vi "FR GUI Measurement setup.vi"(9 "FFmeter settings":T1={"AC Source"={"AC Source type"=enum."Fluke 5XXX calibrator", "VISA"="", "Ref. clock (Hz)"=0.0, "status ref"=refnum}, "TWM pipe"="\\\\.\\pipe\\TWM:server", "Measurement status ref"=refnum, "TWM Status ref"=refnum, "Abort ref"=refnum, "DC meter"={"DC meter type"=enum."H/A/K 3458", "DC meter VISA"="", "NPLC"=10, "status ref"=refnum}, "Measurement properties"={"Measurement frequencies (Hz)"=[1000.0], "Sampling frequency (Hz)"=500000.0, "Signal amplitude (V)"=4.5, "AC-DC settle time (s)"=20.0, "Record length (multiples of period)"=[1000.0, 10000.0, 1000.0], "Measurement template file"=path "", "Row of START keyword"=1, "Row of STOP keyword"=0, "Calculate RMS from samples"=FALSE, "AC-DC warm up time (s)"=300.0, "Measurement template line"=[], "DC meter readings No."=10, "Algorithm"="TWM-WFFT"}, "Skip waiting ref"=refnum, "Octave paths"={"GNU Octave path"=path "C:/Program Files/GNU Octave/Octave-6.2.0/mingw64/bin", "TWM+QWTB path"=path "C:/Users/labina/Desktop/TWM-1.8.7.0-full/octprog", "lvlib path"=path "D:/martin/WAC/WACsw - github/control_software/Filter function meter/external libraries/GOLPI 0.7.3.1 source distribution LV 20.0 32 bit/lv_proc.dll"}, "Template definition"={"Keywords column"=0, "Sig. freq. column"=1, "Rec. len. column"=2, "Meas. points. row min to read"=9, "Meas. points. row max to read"=1509, "Properties column"=4, "Properties row start"=1, "Properties row end"=5, "Keyword START regexp"="", "Keyword STOP regexp"="", "HW data column"=7, "HW data row start"=1, "HW data row end"=3, "TIme and date column start"=3, "Digitizer value column start "=4, "DC mean column start "=6, "DC readings column start"=10}} {"Measurement properties"."Record length (multiples of period)" format="%#_3p"; "Measurement properties"."Sampling frequency (Hz)" format="%#_3p"; "Measurement properties"."Measurement frequencies (Hz)" format="%#_3p"}) -> (3 "FFmeter settings out":T1={"AC Source"={"AC Source type"=enum."Fluke 5XXX calibrator", "VISA"="", "Ref. clock (Hz)"=0.0, "status ref"=refnum}, "TWM pipe"="\\\\.\\pipe\\TWM:server", "Measurement status ref"=refnum, "TWM Status ref"=refnum, "Abort ref"=refnum, "DC meter"={"DC meter type"=enum."H/A/K 3458", "DC meter VISA"="", "NPLC"=10, "status ref"=refnum}, "Measurement properties"={"Measurement frequencies (Hz)"=[1000.0], "Sampling frequency (Hz)"=500000.0, "Signal amplitude (V)"=4.5, "AC-DC settle time (s)"=20.0, "Record length (multiples of period)"=[1000.0, 10000.0, 1000.0], "Measurement template file"=path "", "Row of START keyword"=1, "Row of STOP keyword"=0, "Calculate RMS from samples"=FALSE, "AC-DC warm up time (s)"=300.0, "Measurement template line"=[], "DC meter readings No."=10, "Algorithm"="TWM-WFFT"}, "Skip waiting ref"=refnum, "Octave paths"={"GNU Octave path"=path "C:/Program Files/GNU Octave/Octave-6.2.0/mingw64/bin", "TWM+QWTB path"=path "C:/Users/labina/Desktop/TWM-1.8.7.0-full/octprog", "lvlib path"=path "D:/martin/WAC/WACsw - github/control_software/Filter function meter/external libraries/GOLPI 0.7.3.1 source distribution LV 20.0 32 bit/lv_proc.dll"}, "Template definition"={"Keywords column"=0, "Sig. freq. column"=1, "Rec. len. column"=2, "Meas. points. row min to read"=9, "Meas. points. row max to read"=1509, "Properties column"=4, "Properties row start"=1, "Properties row end"=5, "Keyword START regexp"="", "Keyword STOP regexp"="", "HW data column"=7, "HW data row start"=1, "HW data row end"=3, "TIme and date column start"=3, "Digitizer value column start "=4, "DC mean column start "=6, "DC readings column start"=10}} {"Measurement properties"."Record length (multiples of period)" format="%#_3p"; "Measurement properties"."Sampling frequency (Hz)" format="%#_3p"; "Measurement properties"."Measurement frequencies (Hz)" format="%#_3p"})   [LabVIEW 2020]
uses:
  Type definitions/FFmeter settings.ctl
  General AC source/Type definitions/AC Source.ctl
  General AC source/Type definitions/AC Source type.ctl
  General DC meter/Type definitions/DC meter.ctl
  General DC meter/Type definitions/DC meter type.ctl
  FR Measurement/Type definitions/FR Measuement properties.ctl
  FR Utilities/Type definitions/FR Template definition.ctl
  <vilib>/Utility/error.llb/Error Cluster From Error Code.vi
  <vilib>/ErrorRing/Error Ring.xnode
  external libraries/varilib/varilib.lvlib
panel:
  out "Algorithm":string
  out "dc meter readings":i32=50000 caption="DC meter readings"
  in  "recalculate template":bool
  out "ac-dc warmup time":dbl=50000.0 caption="AC-DC warm-up time" format="%#_6p"
  out "Estimate as formatted text":string
  out "Meas points":i32=1 caption="Measurement points"
  in  "Calculate RMS\nfrom samples":bool
  out "ac-dc settle time":dbl=50000.0 caption="AC-DC settle time" format="%#_6p"
  out "Measurement freq. (Hz) | Record length (periods)":dbl[][](array[numeric])=[[1000.0]] format="%#_3p"
  in  "load template":bool
  in  "Measurement template file":path
  in  "show connections":bool
  out "Signal amplitude (V)":dbl=1.0 caption="AC voltage amplitude"
  out "Sampling frequency (Hz)":dbl=50000.0 caption="Sampling frequency" format="%#_6p"
  out "gui_elements":refnum<vi>[](array[refnum])
  in  "save_and_quit":bool
  in  "cancel":bool
  # "Load the template and check loaded values here:"
  # "s"
  # "V"
  # "Who will make\nnice pictures?\n\nconnection setup here"
  # "Hz"
  # "s"
  # "Who will make\nnice pictures?\n\nwaveforms here"
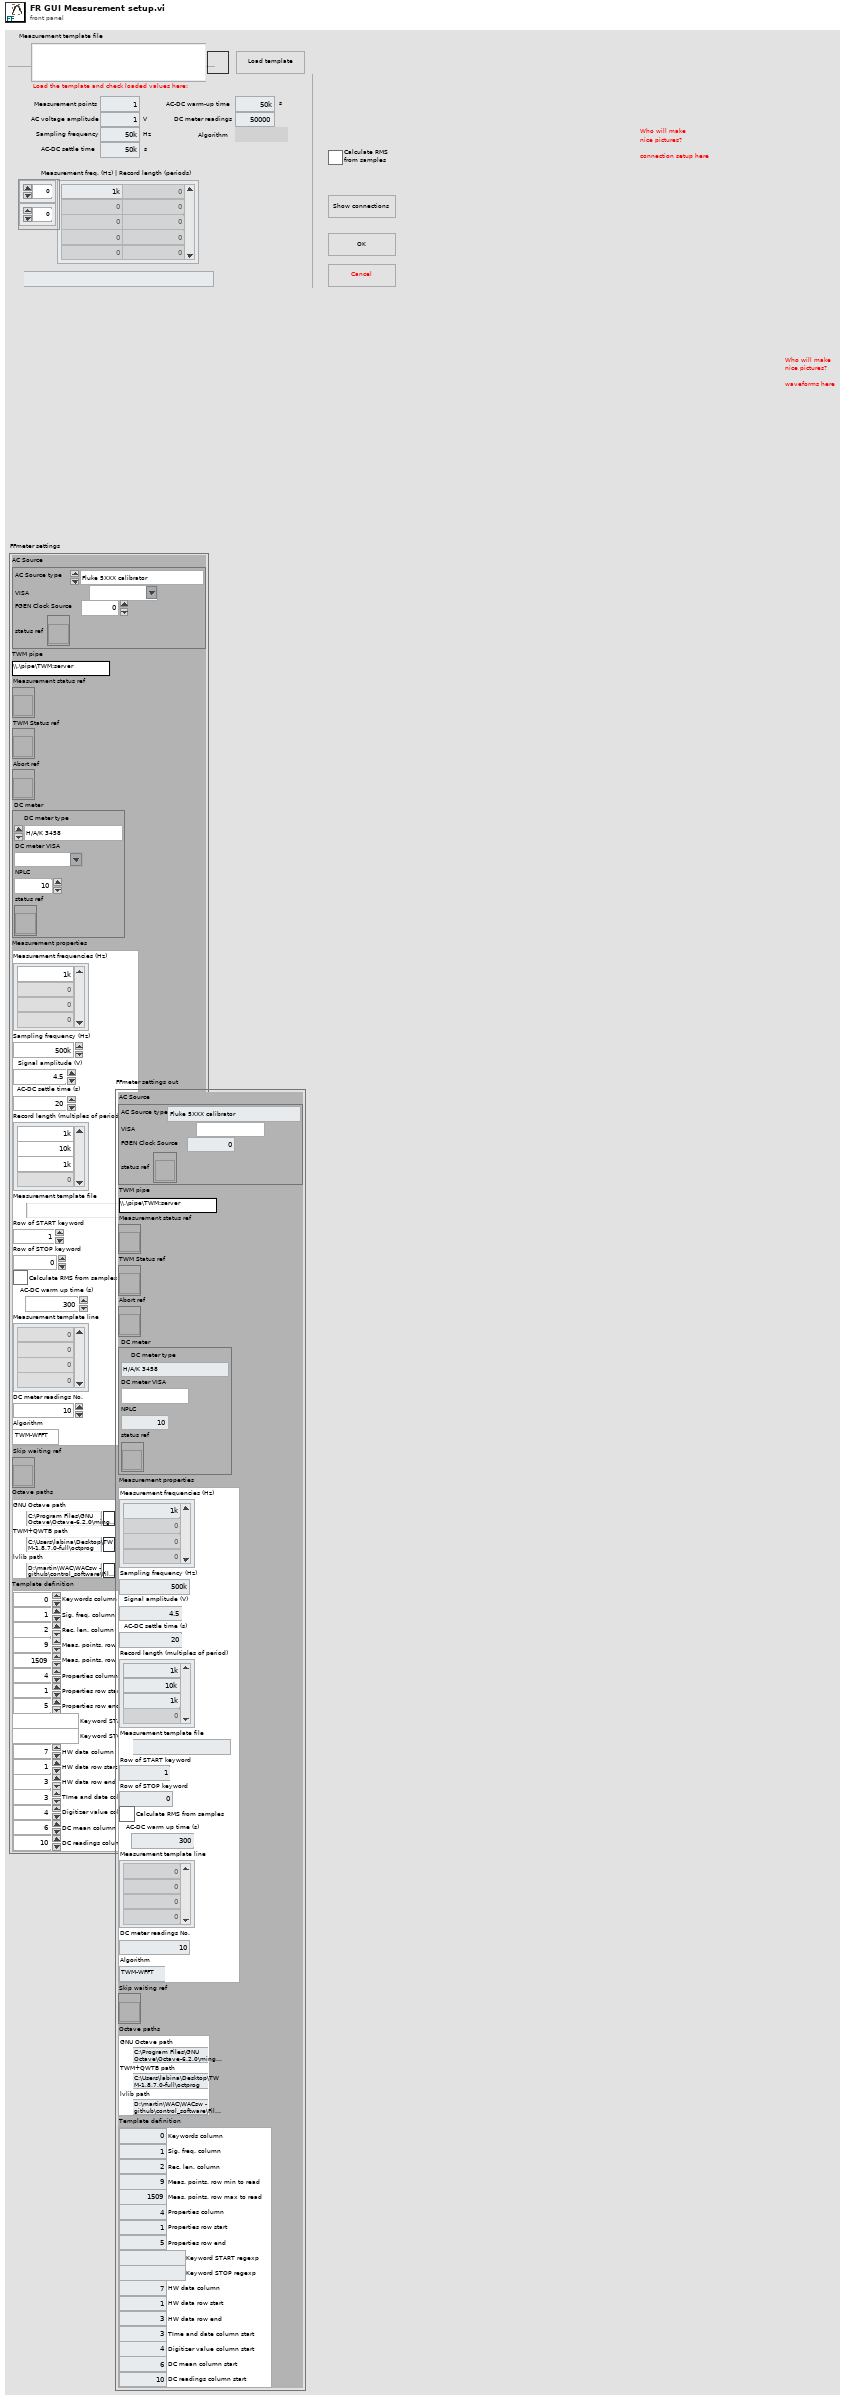
[diagram p1: front panel]
types:
  T1 = typedef "FFmeter settings.ctl" = cluster{"AC Source":T2, "TWM pipe":string, "Measurement status ref":refnum<vi>, "TWM Status ref":refnum<vi>, "Abort ref":refnum<vi>, "DC meter":T4, "Measurement properties":T6, "Skip waiting ref":refnum<vi>, "Octave paths":cluster{"GNU Octave path":path, "TWM+QWTB path":path, "lvlib path":path}, "Template definition":T7}
  T2 = typedef "AC Source.ctl" = cluster{"AC Source type":T3, "VISA":refnum<visa-resource-name>, "Ref. clock (Hz)":dbl, "status ref":refnum<vi>}
  T3 = typedef "AC Source type.ctl" = enum16{"Fluke 5XXX calibrator", "Tektronix AFG3000 series", "dummy"}
  T4 = typedef "DC meter.ctl" = cluster{"DC meter type":T5, "DC meter VISA":refnum<visa-resource-name>, "NPLC":i32, "status ref":refnum<vi>}
  T5 = typedef "DC meter type.ctl" = enum16{"H/A/K 3458", "FLuke 8508A", "dummy"}
  T6 = typedef "FR Measuement properties.ctl" = cluster{"Measurement frequencies (Hz)":dbl[], "Sampling frequency (Hz)":dbl, "Signal amplitude (V)":dbl, "AC-DC settle time (s)":dbl, "Record length (multiples of period)":dbl[], "Measurement template file":path, "Row of START keyword":i32, "Row of STOP keyword":i32, "Calculate RMS from samples":bool, "AC-DC warm up time (s)":dbl, "Measurement template line":i32[], "DC meter readings No.":i32, "Algorithm":string}
  T7 = typedef "FR Template definition.ctl" = cluster{"Keywords column":i32, "Sig. freq. column":i32, "Rec. len. column":i32, "Meas. points. row min to read":i32, "Meas. points. row max to read":i32, "Properties column":i32, "Properties row start":i32, "Properties row end":i32, "Keyword START regexp":string, "Keyword STOP regexp":string, "HW data column":i32, "HW data row start":i32, "HW data row end":i32, "TIme and date column start":i32, "Digitizer value column start ":i32, "DC mean column start ":i32, "DC readings column start":i32}
  T8 = enum32{"Bad", "Idle", "Run top level", "Running"}
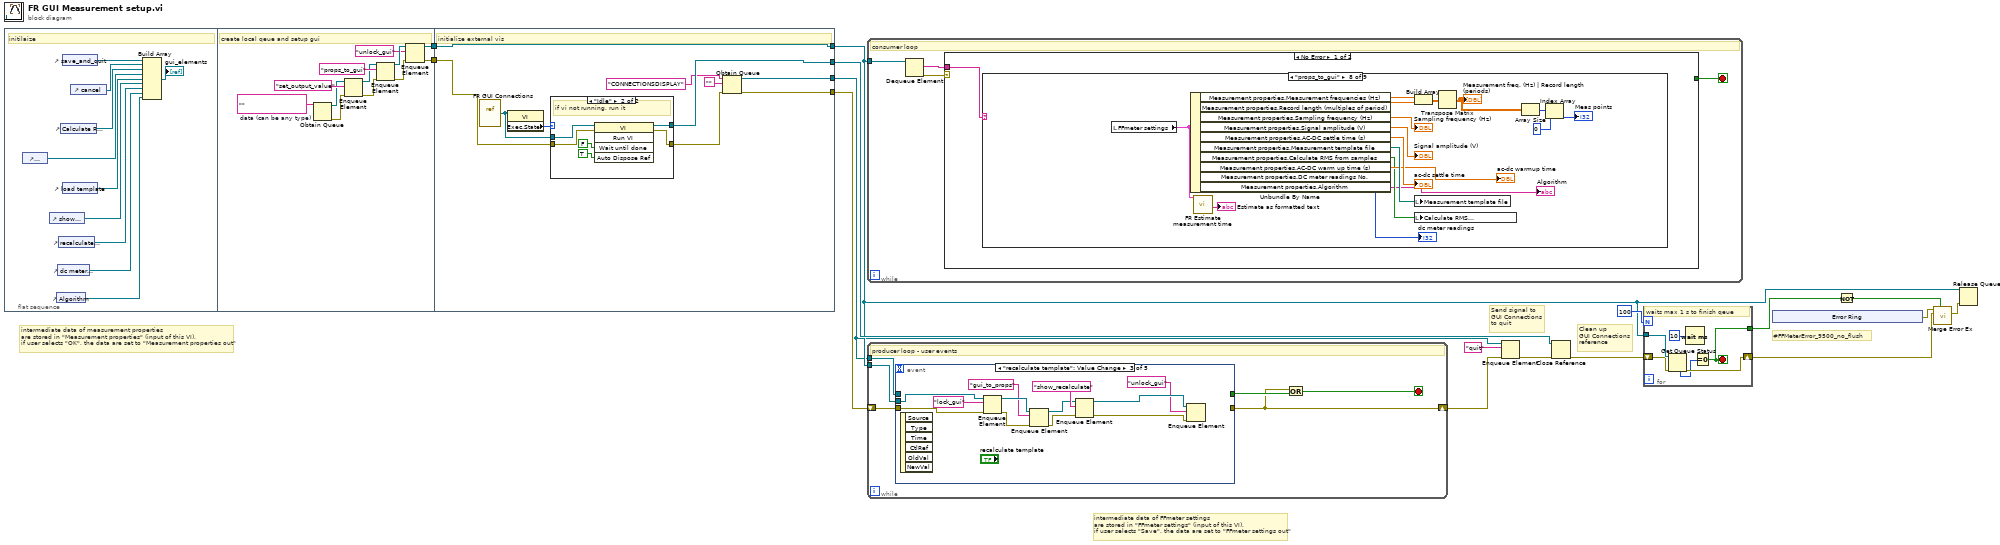
[diagram p0: block diagram]
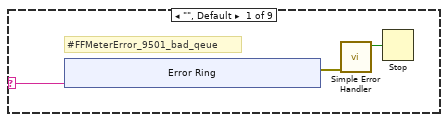
[diagram p3: hidden frame]
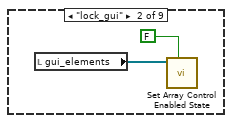
[diagram p4: hidden frame]
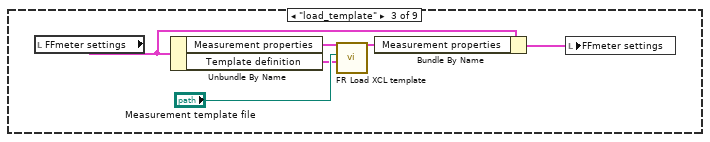
[diagram p5: hidden frame]
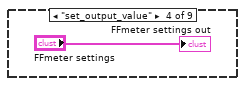
[diagram p6: hidden frame]
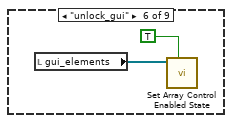
[diagram p8: hidden frame]
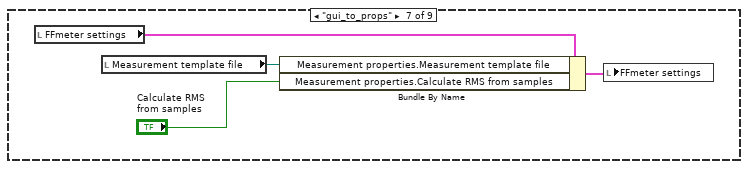
[diagram p9: hidden frame]
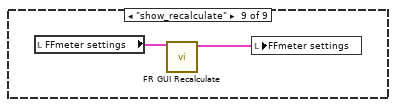
[diagram p10: hidden frame]
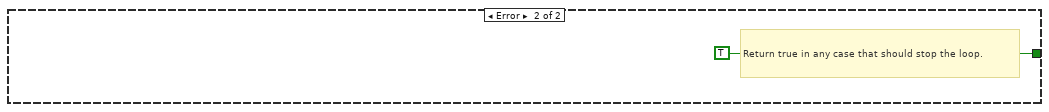
[diagram p11: hidden frame]
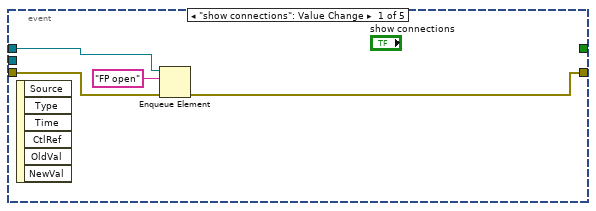
[diagram p12: hidden frame]
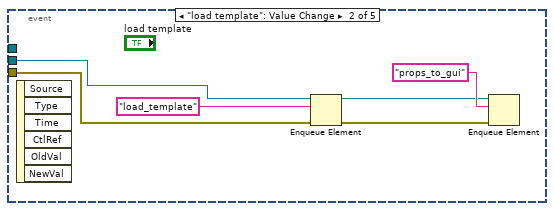
[diagram p13: hidden frame]
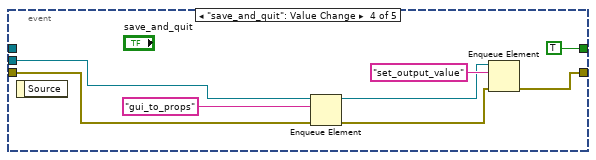
[diagram p14: hidden frame]
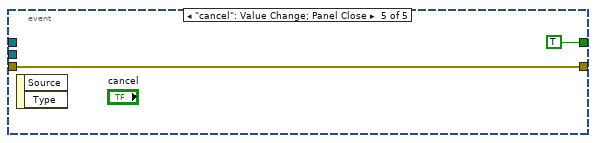
[diagram p15: hidden frame]
diagram:
  # "intermediate data of measurement properties\nare stored in \"Measurement properties\" (input of this VI),\nif user selects \"OK\", the data are set to \"Measurement properties out\""
  # "intermediate data of FFmeter settings\nare stored in \"FFmeter settings\" (input of this VI),\nif user selects \"Save\", the data are set to \"FFmeter settings out\""
  # "Send signal to\nGUI Connections\nto quit"
  # "Clean up\nGUI Connections\nreference"
  # "#FFMeterError_9500_no_flush"
  n1 = flat-sequence {
    tunnel: [w34] -> w9
    tunnel: [w35] -> w8
    tunnel: [w44] -> w10
    tunnel: [w48] -> w3
    tunnel: w9 -> [w48]
    tunnel: w8 -> [w47]
    tunnel: [w45] -> w2
    tunnel: [w46] -> w5
    frame #0 {
      # "initilaize"
      n2 = control-ref of="Measurement template file"() -> (w22:refnum<vi>)
      n3 = control-ref of="show connections"() -> (w20:refnum<vi>)
      n4 = control-ref of="Algorithm"() -> (w17:refnum<vi>)
      n5 = control-ref of="dc meter readings"() -> (w18:refnum<vi>)
      n6 = control-ref of="recalculate template"() -> (w19:refnum<vi>)
      n7 = control-ref of="Calculate RMS\nfrom samples"() -> (w23:refnum<vi>)
      n8 = control-ref of="save_and_quit"() -> (w26:refnum<vi>)
      n9 = control-ref of="load template"() -> (w21:refnum<vi>)
      n10 = control-ref of="cancel"() -> (w25:refnum<vi>)
      n11 = Build Array(w26, w25, w23, w22, w21, w20, w19, w18, w17) -> (→"gui_elements":refnum<vi>[])
    }
    frame #1 {
      w37 = ""  # data (can be any type)
      # "create local qeue and setup gui"
      n12 = Obtain Queue(element data type=w37) -> (queue out=w28:refnum<queue>, error out=w27:errorcluster)  [unwired: 4 in, 1 out]
      n13 = Enqueue Element(queue=w28, element="set_output_value", error in (no error)=w27) -> (queue out=w30:refnum<queue>, error out=w29:errorcluster)  [unwired: 1 in, 1 out]
      n14 = Enqueue Element(queue=w30, element="props_to_gui", error in (no error)=w29) -> (queue out=w33:refnum<queue>, error out=w36:errorcluster)  [unwired: 1 in, 1 out]
      n15 = Enqueue Element(queue=w33, element="unlock_gui", error in (no error)=w36) -> (queue out=w34:refnum<queue>, error out=w35:errorcluster)  [unwired: 1 in, 1 out]
    }
    frame #2 {
      # "initialize external vis"
      n16 = vi-ref "FR GUI Connections.vi"() -> (w42:refnum<vi>)
      n17 = property class="VI"(reference=w42) -> ("Exec.State"=w43:T8)  [unwired: 1 in, 2 out]
      n18 = case shown="\"Idle\"" w43 {
        tunnel: [w49 w56] -> w39
        tunnel: w47 -> [w49 w53]
        tunnel: [w50 w52] -> w46
        tunnel: w42 -> [w50 w51]
        frame "Bad", Default {
        }
        frame "Idle" {
          # "if vi not running, run it"
          n19 = invoke class="VI" method="Run VI"(reference=w51, error in=w53, "Wait until done"=FALSE ("Wait Until Done"), "Auto Dispose Ref"=TRUE ("Wait Until Done")) -> (reference out=w52:refnum<vi>, error out=w56:errorcluster)  [unwired: 1 in, 3 out]
        }
      }
      n20 = Obtain Queue(name (unnamed)="CONNECTIONSDISPLAY", element data type="", error in (no error)=w39) -> (queue out=w45:refnum<queue>, error out=w44:errorcluster)  [unwired: 2 in, 1 out]
    }
  }
  n21 = while {
    tunnel: w3 -> [w60]
    stop <- w57 stop-if-true
    # "consumer loop"
    n22 = Dequeue Element(queue=w60) -> (element=w58:string, error out=w59:errorcluster)  [unwired: 2 in, 2 out]
    n23 = case shown="No Error" w59 {
      tunnel: w58 -> [w61 _]
      tunnel: [_ TRUE] -> w57
      frame No Error {
        n24 = case shown="\"props_to_gui\"" w61 {
          selector: w61 -> [w62 _ _ _ _ _ _ _ _]
          frame "", Default {
            # "#FFMeterError_9501_bad_qeue"
            n25 = xnode "Error Ring"("parameter 0"=w62) -> ("error out"=w64:errorcluster)
            n26 = call <vilib>:"Simple Error Handler.vi"("error in (no error)"=w64) -> ("error?"=w63:bool)  [unwired: 4 in, 4 out]
            n27 = Stop(stop? (T)=w63) -> ()
          }
          frame "lock_gui" {
            n28 = local read "gui_elements"() -> (w73:refnum<vi>[])
            n29 = call "Set Array Control Enabled State.vi"("enabled (T)"=FALSE, "reference array in"=w73) -> ()  [unwired: 8 in, 2 out]
          }
          frame "load_template" {
            n30 = local read "FFmeter settings"() -> (w77:T1)
            n31 = Unbundle By Name(w77) -> ("Measurement properties"=w76:T6, "Template definition"=w74:T7)
            n32 = call "FR Load XCL template.vi"("Template definition"=w74, "Measurement template file"="Measurement template file", "Measurement properties"=w76) -> ("Measurement properties out"=w75:T6)  [unwired: 8 in]
            n33 = Bundle By Name(cluster=w77, "Measurement properties"=w75) -> (w78:T1)
            n34 = local write "FFmeter settings"(w78) -> ()
          }
          frame "set_output_value" {
            "FFmeter settings out" <- "FFmeter settings"
          }
          frame "create_template" {
          }
          frame "unlock_gui" {
            n35 = local read "gui_elements"() -> (w82:refnum<vi>[])
            n36 = call "Set Array Control Enabled State.vi"("enabled (T)"=TRUE, "reference array in"=w82) -> ()  [unwired: 8 in, 2 out]
          }
          frame "gui_to_props" {
            n37 = local read "FFmeter settings"() -> (w85:T1)
            n38 = local read "Measurement template file"() -> (w83:path)
            n39 = Bundle By Name(cluster=w85, "Measurement properties.Measurement template file"=w83, "Measurement properties.Calculate RMS from samples"="Calculate RMS\nfrom samples") -> (w86:T1)
            n40 = local write "FFmeter settings"(w86) -> ()
          }
          frame "props_to_gui" {
            n41 = local read "FFmeter settings"() -> (w92:T1)
            n42 = Unbundle By Name(w92) -> ("Measurement properties.Measurement frequencies (Hz)"=w103:dbl[], "Measurement properties.Record length (multiples of period)"=w102:dbl[], "Measurement properties.Sampling frequency (Hz)"=→"Sampling frequency (Hz)":dbl, "Measurement properties.Signal amplitude (V)"=→"Signal amplitude (V)":dbl, "Measurement properties.AC-DC settle time (s)"=→"ac-dc settle time":dbl, "Measurement properties.Measurement template file"=w99:path, "Measurement properties.Calculate RMS from samples"=w88:bool, "Measurement properties.AC-DC warm up time (s)"=→"ac-dc warmup time":dbl, "Measurement properties.DC meter readings No."=→"dc meter readings":i32, "Measurement properties.Algorithm"=→"Algorithm":string)
            n43 = call "FR Estimate measurement time.vi"("FFmeter settings"=w92) -> ("Estimate as formatted text"=→"Estimate as formatted text":string)  [unwired: 9 in, 1 out]
            n44 = Build Array(w103, w102) -> (w97:dbl[][])
            n45 = local write "Measurement template file"(w99) -> ()
            n46 = local write "Calculate RMS\nfrom samples"(w88) -> ()
            n47 = Transpose Matrix(1:w97) -> (0:w96:dbl[][])
            "Measurement freq. (Hz) | Record length (periods)" <- w96
            n48 = Array Size(array=w96) -> (size(s)=w95:i32[])
            n49 = Index Array(array=w95, index=0) -> (element=→"Meas points":i32)
          }
          frame "show_recalculate" {
            n50 = local read "FFmeter settings"() -> (w105:T1)
            n51 = call "FR GUI Recalculate.vi"("FFmeter settings"=w105) -> ("FFmeter settings out"=w104:T1)  [unwired: 10 in]
            n52 = local write "FFmeter settings"(w104) -> ()
          }
        }
      }
      frame Error {
        # "Return true in any case that should stop the loop."
      }
    }
  }
  n53 = while {
    shift-right: [w108] -> w4
    shift-left: w10 -> [w111]
    tunnel: w3 -> [w112]
    tunnel: w2 -> [w107]
    stop <- w109 stop-if-true
    # "producer loop - user events"
    n54 = event shown="[2] \"recalculate template\": Value Change" {
      selector: _ -> [_ _ _ _ _]
      dyn-events: _ -> [_ _ _ _ _]
      timeout: _ -> [_ _ _ _ _]
      tunnel: w112 -> [_ w121 w129 w141 _]
      tunnel: w111 -> [w115 w120 w130 w140 w143]
      tunnel: [w114 _ _ w138 w143] -> w108
      tunnel: [_ _ _ TRUE ("cancel") TRUE ("cancel")] -> w110
      tunnel: w107 -> [w113 _ _ _ _]
      event "show connections": Value Change {
        n55 = event-data() -> ()  [unwired: 1 in, 6 out]
        n56 = Enqueue Element(queue=w113, element="FP open", error in (no error)=w115) -> (error out=w114:errorcluster)  [unwired: 1 in, 2 out]
      }
      event "load template": Value Change {
        n57 = event-data() -> ()  [unwired: 1 in, 6 out]
        n58 = Enqueue Element(queue=w121, element="load_template", error in (no error)=w120) -> (queue out=w117:refnum<queue>, error out=w119:errorcluster)  [unwired: 1 in, 1 out]
        n59 = Enqueue Element(queue=w117, element="props_to_gui", error in (no error)=w119) -> ()  [unwired: 1 in, 3 out]
      }
      event "recalculate template": Value Change {
        n60 = event-data() -> ()  [unwired: 1 in, 6 out]
        n61 = Enqueue Element(queue=w129, element="lock_gui", error in (no error)=w130) -> (queue out=w124:refnum<queue>, error out=w127:errorcluster)  [unwired: 1 in, 1 out]
        n62 = Enqueue Element(queue=w124, element="gui_to_props", error in (no error)=w127) -> (queue out=w125:refnum<queue>, error out=w126:errorcluster)  [unwired: 1 in, 1 out]
        n63 = Enqueue Element(queue=w125, element="show_recalculate", error in (no error)=w126) -> (queue out=w132:refnum<queue>, error out=w133:errorcluster)  [unwired: 1 in, 1 out]
        n64 = Enqueue Element(queue=w132, element="unlock_gui", error in (no error)=w133) -> ()  [unwired: 1 in, 3 out]
      }
      event "save_and_quit": Value Change {
        n65 = event-data() -> ()  [unwired: 1 in, 1 out]
        n66 = Enqueue Element(queue=w141, element="gui_to_props", error in (no error)=w140) -> (queue out=w135:refnum<queue>, error out=w139:errorcluster)  [unwired: 1 in, 1 out]
        n67 = Enqueue Element(queue=w135, element="set_output_value", error in (no error)=w139) -> (error out=w138:errorcluster)  [unwired: 1 in, 2 out]
      }
      event "cancel": Value Change; Panel Close {
        n68 = event-data() -> ()  [unwired: 1 in, 2 out]
      }
    }
    n69 = Or(x=w108, y=w110) -> (x .or. y?=w109:bool)
  }
  n70 = Enqueue Element(queue=w2, element="quit", error in (no error)=w4) -> (error out=w7:errorcluster)  [unwired: 1 in, 2 out]
  n71 = Close Reference(reference=w5, error in (no error)=w7) -> (error out=w1:errorcluster)
  n72 = for {
    N: 100 -> [_]
    tunnel: w3 -> [w150]
    shift-right: [w148] -> w13
    shift-left: w1 -> [w149]
    tunnel: [w145] -> w11
    stop <- w145 stop-if-true
    # "waits max 1 s to finish qeue"
    n73 = Get Queue Status(queue=w150, error in (no error)=w149) -> (error out=w148:errorcluster, # elements in queue=w146:i32)  [unwired: 1 in, 6 out]
    n74 = Wait (ms)(milliseconds to wait=u32 10) -> ()  [unwired: 1 out]
    n75 = Equal To 0?(x=w146) -> (x = 0?=w145:bool)
  }
  n76 = xnode "Error Ring"() -> ("error out"=w14:errorcluster)
  n77 = Not(x=w11) -> (.not. x?=w15:bool)
  n78 = call "Merge Error Ex.vi"("Is error? (False)"=w15, "main error in (no error)"=w13, "second error in"=w14) -> ("error out"=w12:errorcluster)  [unwired: 8 in]
  n79 = Release Queue(queue=w3, error in (no error)=w12) -> ()  [unwired: 1 in, 3 out]
